vi "medidorIXV.vi"(7 "Ponto":i32) -> (1 "Array":dbl[](array[numeric]), 2 "Corrente Atual":dbl, 3 "Tensao Atual":dbl)   [LabVIEW 2012]
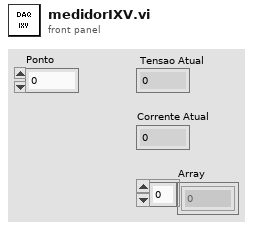
[diagram p1: front panel]
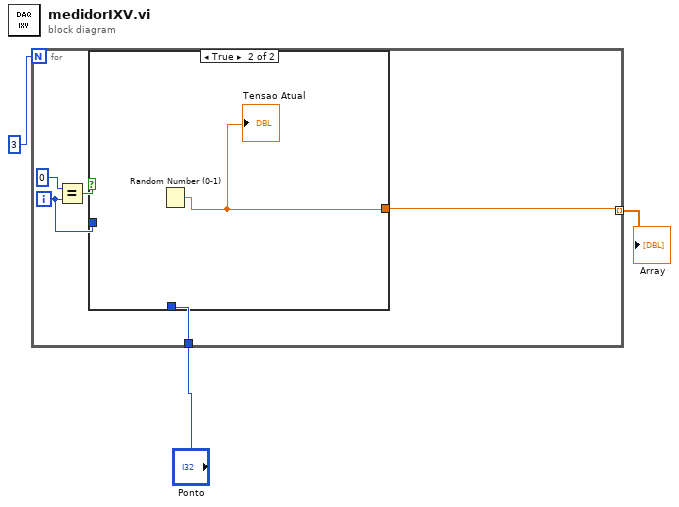
[diagram p0: block diagram]
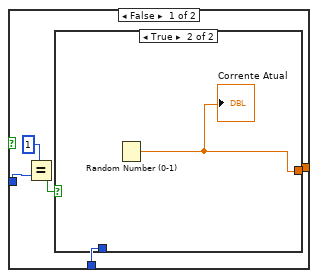
[diagram p2: hidden frame]
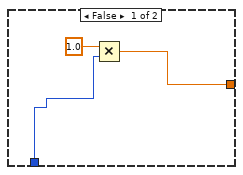
[diagram p3: hidden frame]
diagram:
  n1 = for {
    N: 3 -> [_]
    tunnel: [w5] -> w1 mode=indexing
    tunnel: "Ponto" -> [w4]
    i -> [w6]
    n2 = Equal?(x=0, y=w6) -> (x = y?=w7:bool)
    n3 = case shown="True" w7 {
      tunnel: [w9 w18] -> w5
      tunnel: w6 -> [w12 _]
      tunnel: w4 -> [w10 _]
      frame False {
        n4 = Equal?(x=1, y=w12) -> (x = y?=w11:bool)
        n5 = case shown="True" w11 {
          tunnel: w10 -> [w14 _]
          tunnel: [w16 w17] -> w9
          frame False {
            n6 = Multiply(x=1.0, y=w14) -> (x*y=w16:dbl)
          }
          frame True {
            n7 = Random Number (0-1)() -> (number: 0 to 1=w17:dbl)
            "Corrente Atual" <- w17
          }
        }
      }
      frame True {
        n8 = Random Number (0-1)() -> (number: 0 to 1=w18:dbl)
        "Tensao Atual" <- w18
      }
    }
  }
  "Array" <- w1
